vi "Write TDMS.vi"(8 "error in (no error)":errorcluster, 10 "path":path, 11 "LVtoITX in":refnum<class "LVtoITX.lvclass">) -> (0 "error out":errorcluster, 3 "LVtoITX out":refnum<class "LVtoITX.lvclass">)   [LabVIEW 2016, in "LVtoITX.lvclass"]
uses:
  LVtoITX.lvclass
  LVtoITX.lvclass/LVtoITX.ctl
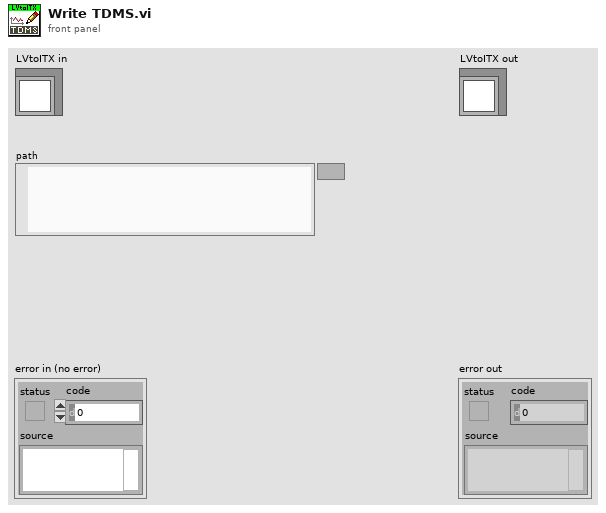
[diagram p1: front panel]
types:
  T1 = enum16{"open", "open or create", "create or replace", "create", "open (read-only)"}
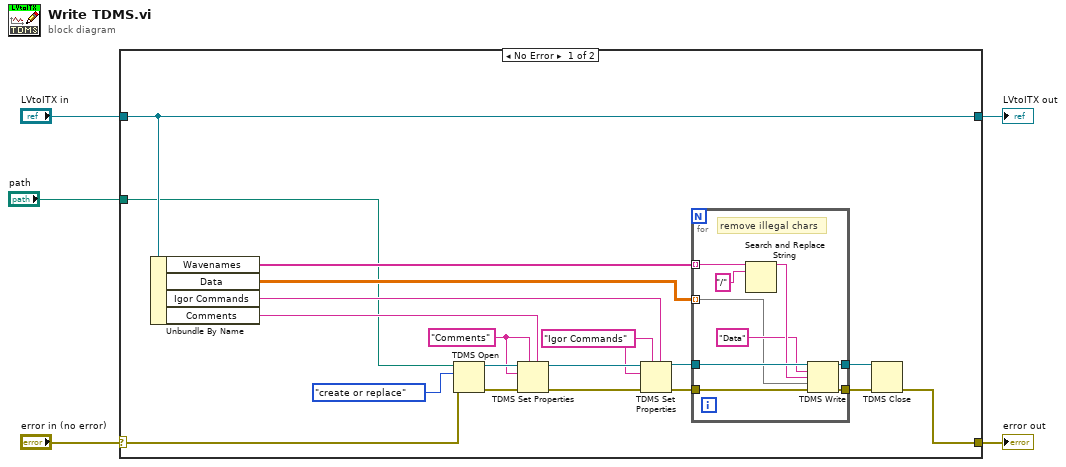
[diagram p0: block diagram]
diagram:
  n1 = case shown="No Error" "error in (no error)" {
    selector: "error in (no error)" -> [w12 w34]
    tunnel: [w16 w34] -> w2
    tunnel: [w24 w35] -> w3
    tunnel: "LVtoITX in" -> [w24 w35]
    tunnel: "path" -> [w8 _]
    frame No Error {
      w7 = "Igor Commands" ("attrib name")
      w6 = "Comments" ("attrib name")
      n2 = Unbundle By Name(w24) -> ("Wavenames"=w11:string[], "Data"=w10:dbl[][], "Igor Commands"=w13:string, "Comments"=w14:string)
      n3 = TDMS Open(8:w12, 10:T1."create or replace" ("operation (0:open)"), 11:w8) -> (0:w23:errorcluster, 3:w22:refnum<k34>)  [unwired: 4 in]
      n4 = TDMS Set Properties(5:w14, 7:w6, 8:w23, 10:w6, 11:w22) -> (0:w20:errorcluster, 3:w21:refnum<k34>)  [unwired: 1 in, 2 out]
      n5 = TDMS Set Properties(5:w13, 7:w7, 8:w20, 10:w7, 11:w21) -> (0:w19:errorcluster, 3:w18:refnum<k34>)  [unwired: 1 in, 2 out]
      n6 = for {
        tunnel: w11 -> [w33] mode=indexing
        tunnel: w10 -> [w25] mode=indexing
        tunnel: w19 -> [w31]
        tunnel: w18 -> [w30]
        tunnel: [w29] -> w17
        tunnel: [w28] -> w15
        # "remove illegal chars"
        n7 = Search and Replace String(input string=w33, search string="/") -> (result string=w27:string)  [unwired: 6 in, 3 out]
        n8 = TDMS Write(0:w30, 5:"Data" ("group name in (Untitled)"), 7:w27, 9:w25, 11:w31) -> (4:w28:refnum<k34>, 15:w29:errorcluster)  [unwired: 1 in, 2 out]
      }
      n9 = TDMS Close(8:w17, 11:w15) -> (0:w16:errorcluster)  [unwired: 1 out]
    }
    frame Error {
    }
  }
  "error out" <- w2
  "LVtoITX out" <- w3
